vi "MGCC_FntStaMach_Closeall.vi"   [LabVIEW 2016]
doc: "-----------------------------------------------------------------------------------------------------------------------\nCopyright <2019> <The University of Tennessee at Knoxville and the University of Tennessee Research Foundation>\nThis software is released under BSD-3 \nhttps://opensource.org/licenses/BSD-3-Clause \nAdditional license options available at https://utrf.tennessee.edu/industry/sample-agreements/\n-----------------------------------------------------------------------------------------------------------------------"
uses:
  Communication/Global communication output.vi
  Model Management/Global_MdlMgmt.vi
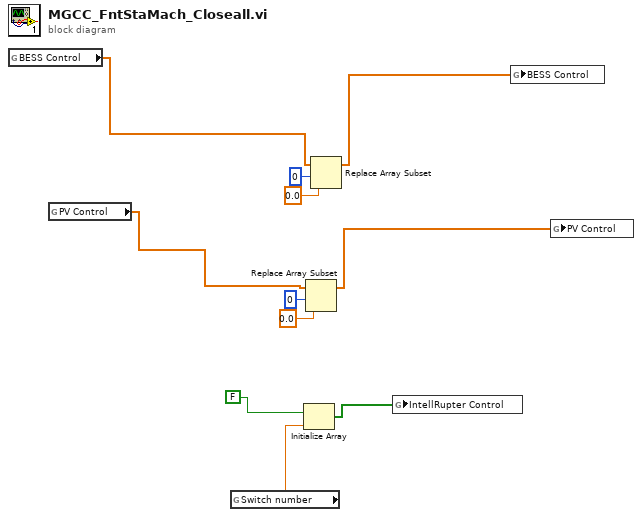
[diagram p0: block diagram]
diagram:
  n1 = global read "Global communication output.vi" "BESS Control"() -> (w7:dbl[])
  n2 = global read "Global communication output.vi" "PV Control"() -> (w6:dbl[])
  n3 = global read "Global_MdlMgmt.vi" "Switch number"() -> (w1:dbl)
  n4 = Initialize Array(FALSE, w1) -> (w2:bool[])
  n5 = Replace Array Subset(array=w6, new element=0.0 ("new element/subarray"), index=0) -> (w4:dbl[])
  n6 = Replace Array Subset(array=w7, new element=0.0 ("new element/subarray"), index=0) -> (w5:dbl[])
  n7 = global write "Global communication output.vi" "IntellRupter Control"(w2) -> ()
  n8 = global write "Global communication output.vi" "BESS Control"(w5) -> ()
  n9 = global write "Global communication output.vi" "PV Control"(w4) -> ()
